vi "STM Write Message (UDP).vi"(4 "Address":cluster{"address":u32, "port":u16}, 6 "Options":T1={"Ignore Timeout Error"=TRUE, "timeout ms (1000)"=1000}, 8 "error in (no error)":errorcluster, 9 "Data":string, 10 "Name":string, 11 "Connection Info":T2) -> (0 "error out":errorcluster, 3 "Connection Info Out":T2)   [LabVIEW 2014, in "QwaveSys Raspberry Pi Library.lvlib"]
doc: "This VI writes a package of data to a remote computer. It prepends a meta data ID number to each packet. \n\nThe data must be passed in as a String. The calling VI is responsible for flattening the desired data to a string before passing it to this VI."
uses:
  QwaveSys Raspberry Pi Library.lvlib
  stm_UDP Connection Info.ctl
  _SubVIs/stm_MetaDataElement.ctl
  stm_UDP Write Options.ctl
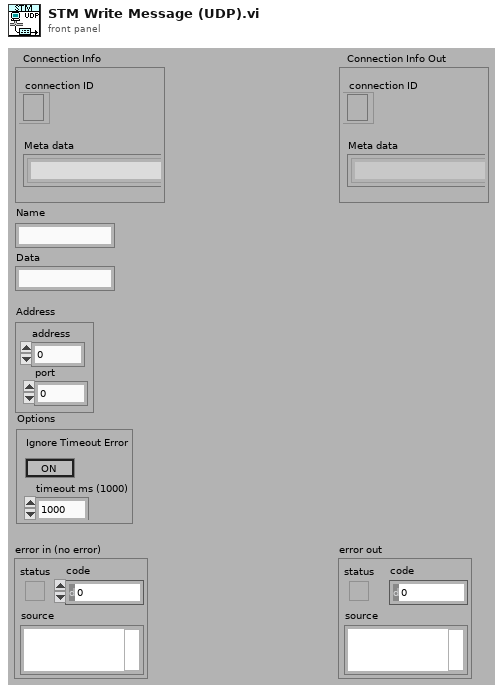
[diagram p1: front panel]
types:
  T1 = typedef "QwaveSys Raspberry Pi Library.lvlib/stm_UDP Write Options.ctl" = cluster{"Ignore Timeout Error":bool, "timeout ms (1000)":i32}
  T2 = typedef "QwaveSys Raspberry Pi Library.lvlib/stm_UDP Connection Info.ctl" = cluster{"connection ID":refnum<k16>, "Meta data":T3[]}
  T3 = typedef "QwaveSys Raspberry Pi Library.lvlib/stm_MetaDataElement.ctl" = string
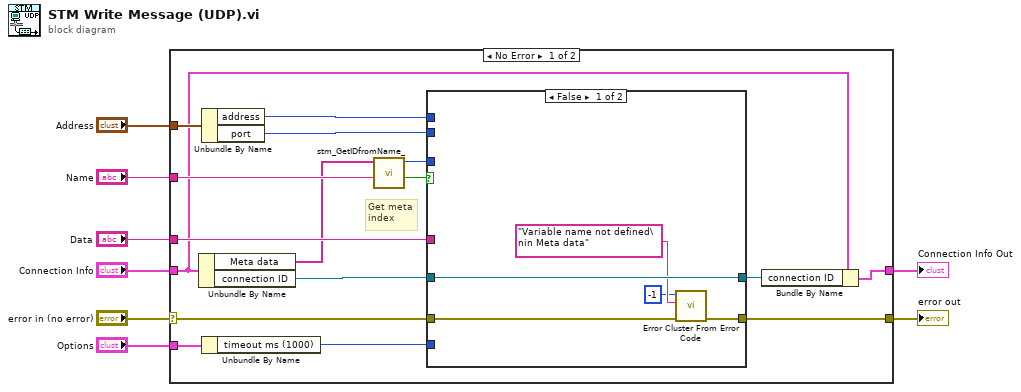
[diagram p0: block diagram]
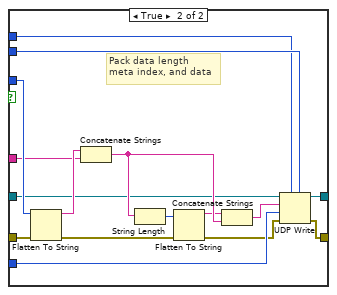
[diagram p2: hidden frame]
diagram:
  n1 = case shown="No Error" "error in (no error)" {
    selector: "error in (no error)" -> [w19 w47]
    tunnel: "Connection Info" -> [w11 w46]
    tunnel: [w24 w47] -> w8
    tunnel: [w9 w46] -> w3
    tunnel: "Name" -> [w23 _]
    tunnel: "Data" -> [w21 _]
    tunnel: "Address" -> [w16 _]
    tunnel: "Options" -> [w13 _]
    frame No Error {
      # "Get meta\nindex"
      n2 = Unbundle By Name(w11) -> ("Meta data"=w14:T3[], "connection ID"=w15:refnum<k16>)
      n3 = Unbundle By Name(w16) -> ("address"=w18:u32, "port"=w17:u16)
      n4 = Unbundle By Name(w13) -> ("timeout ms (1000)"=w12:i32)
      n5 = call "stm_GetIDfromName_.vi"("Name"=w23, "MetaData"=w14) -> ("Found"=w20:bool, "Meta ID"=w22:u16)  [unwired: 8 out]
      n6 = case shown="False" w20 {
        tunnel: w15 -> [w29 w37]
        tunnel: w19 -> [w28 w32]
        tunnel: [w27 w38] -> w24
        tunnel: [w29 w39] -> w10
        tunnel: w22 -> [_ w45]
        tunnel: w21 -> [_ w41]
        tunnel: w18 -> [_ w34]
        tunnel: w17 -> [_ w35]
        tunnel: w12 -> [_ w33]
        frame False {
          n7 = call <vilib>:"Error Cluster From Error Code.vi"("error in (no error)"=w28, "error message (\"\")"="Variable name not defined\nin Meta data" ("source"), "error code (0)"=-1) -> ("error out"=w27:errorcluster)  [unwired: 1 in, 5 out]
        }
        frame True {
          # "Pack data length\nmeta index, and data"
          n8 = Flatten To String(anything=w45, error in (no error)=w32) -> (data string=w44:string, error out=w31:errorcluster)  [unwired: 1 in, 2 out]
          n9 = Concatenate Strings(w44, w41) -> (w42:string)
          n10 = String Length(string=w42) -> (length=w43:i32)
          n11 = Flatten To String(anything=w43, error in (no error)=w31) -> (data string=w40:string, error out=w30:errorcluster)  [unwired: 3 out]
          n12 = Concatenate Strings(w40, w42) -> (w36:string)
          n13 = UDP Write(address=w34, port or service name=w35, connection ID=w37, data in=w36, 8:w30, 9:w33) -> (error out=w38:errorcluster, 3:w39:refnum<k16>)
        }
      }
      n14 = Bundle By Name(cluster=w11, "connection ID"=w10) -> (w9:T2)
    }
    frame Error {
    }
  }
  "error out" <- w8
  "Connection Info Out" <- w3
